vi "Build Reports for Files and Folders.vi"(0 "directory info":T1={"target dir"=path "C:/ADIBitbucket/nists19.0_templateproject/Code Modules/Common/Instrument Control/DCPower", "output dir"={"base dir"=path "../docs", "image dir"=path "../docs", "html dir"=path "../docs", "md dir"=path "../docs"}, "folder names"=[], "filenames"=[]}, 7 "Initial Call":bool, 11 "error in":errorcluster) -> (15 "error out":errorcluster)   [LabVIEW 2019, in "MD Generator.lvlib"]
uses:
  MD Generator.lvlib
  Report Path Cluster.ctl
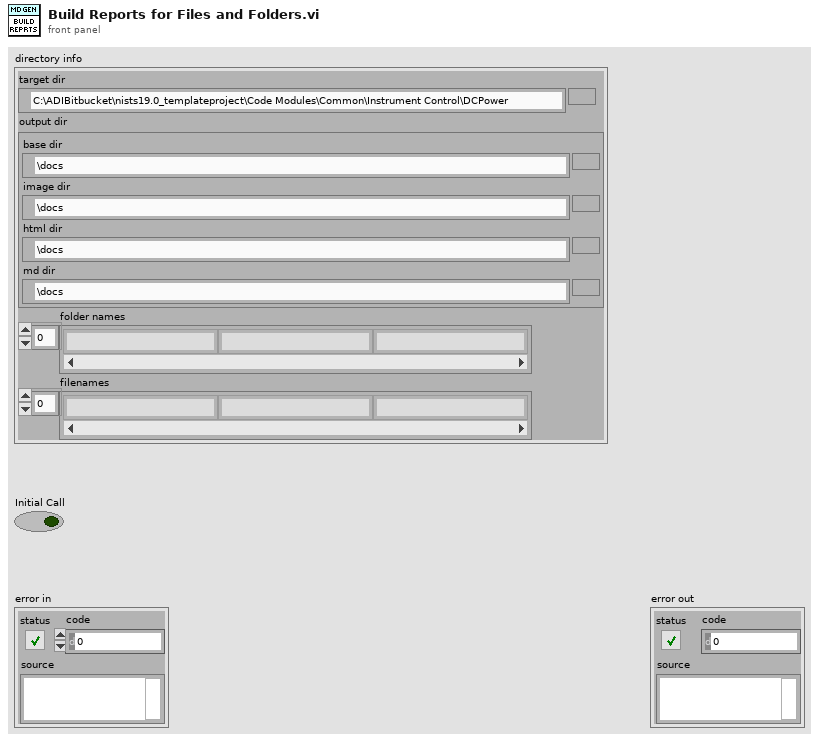
[diagram p1: front panel]
types:
  T1 = typedef "Report Path Cluster.ctl" = cluster{"target dir":path, "output dir":cluster{"base dir":path, "image dir":path, "html dir":path, "md dir":path}, "folder names":string[], "filenames":string[]}
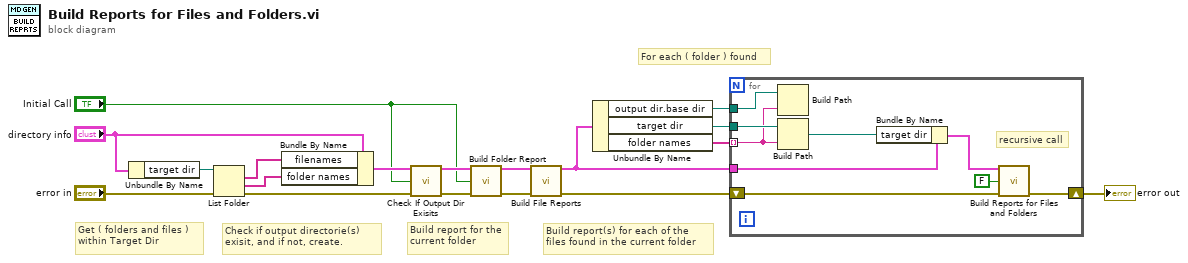
[diagram p0: block diagram]
diagram:
  # "For each ( folder ) found"
  # "Check if output directorie(s) exisit, and if not, create."
  # "Get ( folders and files ) within Target Dir"
  # "Build report for the current folder"
  # "Build report(s) for each of the files found in the current folder"
  n1 = Unbundle By Name("directory info") -> ("target dir"=w12:path)
  n2 = List Folder(path=w12, error in="error in") -> (filenames=w14:string[], folder names=w15:string[], error out=w11:errorcluster)  [unwired: 2 in, 1 out]
  n3 = Bundle By Name(cluster="directory info", "filenames"=w14, "folder names"=w15) -> (w8:T1)
  n4 = call "Check If Output Dir Exisits.vi"("directory info in"=w8, "Initial Call"="Initial Call", "error in"=w11) -> ("directory info out"=w9:T1, "error out"=w10:errorcluster)  [unwired: 11 in]
  n5 = call "Build Folder Report.vi"("directory info in"=w9, "Initial Call"="Initial Call", "error in"=w10) -> ("directory info out"=w17:T1, "error out"=w16:errorcluster)  [unwired: 11 in]
  n6 = call "Build File Reports.vi"("directory info in"=w17, "error in"=w16) -> ("directory info out"=w3:T1, "error out"=w6:errorcluster)  [unwired: 12 in]
  n7 = Unbundle By Name(w3) -> ("output dir.base dir"=w2:path, "target dir"=w4:path, "folder names"=w5:string[])
  n8 = for {
    shift-right: [w26] -> w7
    shift-left: w6 -> [w27]
    tunnel: w4 -> [w25]
    tunnel: w5 -> [w20] mode=indexing
    tunnel: w3 -> [w23]
    tunnel: w2 -> [w21]
    # "recursive call"
    n9 = Build Path(base path=w21, name or relative path=w20) -> ()  [unwired: 1 out]
    n10 = Build Path(base path=w25, name or relative path=w20) -> (appended path=w24:path)
    n11 = Bundle By Name(cluster=w23, "target dir"=w24) -> (w22:T1)
    n12 = call "Build Reports for Files and Folders.vi"("directory info"=w22, "Initial Call"=FALSE, "error in"=w27) -> ("error out"=w26:errorcluster)  [unwired: 12 in]
  }
  "error out" <- w7
